vi "gblV.vi"() -> ()   [LabVIEW 2020]
panel:
  in  "sts":string
  out "Seek":i32
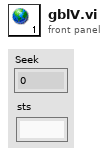
[diagram p1: front panel]
diagram:
